vi "AddTwoNumbersInArray.vi"(3 "Numeric 2":dbl, 4 "Numeric 1":dbl, 5 "Array In":refnum<k24>[](array[refnum])) -> (0 "error out":errorcluster, 1 "Sum":dbl, 2 "Array Out":refnum<k24>[](array[refnum]))   [LabVIEW 2011]
uses:
  D:/tsdev/Tests/LVBuildValidation/11.0/Automated/FlexLVAdapter30/Refnums/DotNetRefnum/LabviewDNTest.dll
  LabviewDNTest.dll
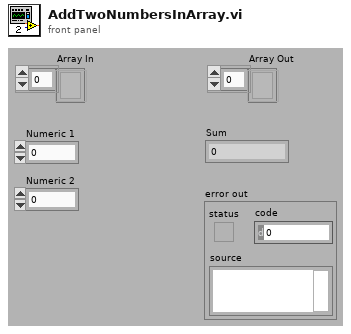
[diagram p1: front panel]
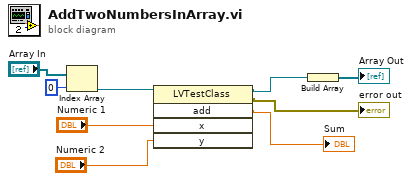
[diagram p0: block diagram]
diagram:
  n1 = Index Array(array="Array In", index=0) -> (element=w6:refnum<k24>)
  n2 = invoke class="LVTestClass" method="add"(reference=w6, "x"="Numeric 1", "y"="Numeric 2") -> (reference out=w1:refnum<k24>, error out=→"error out":errorcluster, "add"=→"Sum":dbl)  [unwired: 2 in, 2 out]
  n3 = Build Array(w1) -> (→"Array Out":refnum<k24>[])
